vi "transition.vi"(8 "error in (no error)":errorcluster, 10 "Context In":refnum<class "Context.lvclass">, 11 "Run in":refnum<class "User State 1.lvclass">) -> (0 "error out":errorcluster, 2 "Context Out":refnum<class "Context.lvclass">, 3 "Run out":refnum<class "User State 1.lvclass">)   [LabVIEW 2018, in "User State 1.lvclass"]
uses:
  User State 1.lvclass
  Context/Context.lvclass
  Wait Event/Wait Event.lvclass
  C:/Users/fflores/Documents/OOP-State-Machine/State/State.lvclass
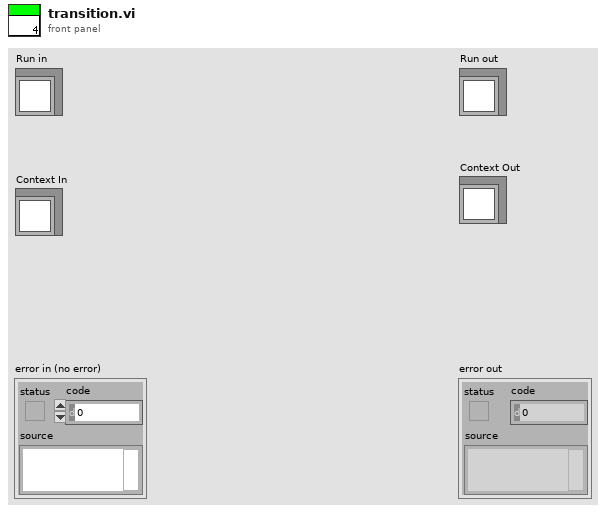
[diagram p1: front panel]
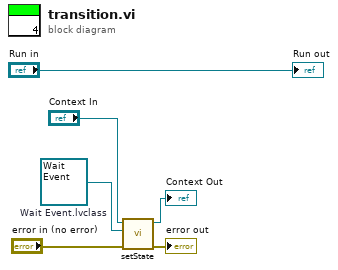
[diagram p0: block diagram]
diagram:
  w1 = refnum<class "Wait Event.lvclass"> refnum  # Wait Event.lvclass
  n1 = call "setState.vi"("error in (no error)"="error in (no error)", "State.lvclass"=w1, "Context in"="Context In") -> ("error out"=→"error out":errorcluster, "Context out"=→"Context Out":refnum<class "Context.lvclass">)  [unwired: 7 in]
  "Run out" <- "Run in"
